vi "Bitte Warten.vi"() -> ()   [LabVIEW 2020, in "allgemeine Sub-VIs.lvlib"]
uses:
  allgemeine Sub-VIs.lvlib
  Visualisierungs Elemente/Button.ctl
  Aktionen Daten am cRIO speichern.ctl
  Sprachverwaltung/FGV Aktion Tabelle zerlegen.ctl
  SysLog/SysLog Interface.ctl
  SysLog/Aktionen FGV SysLog.ctl
  Sprachverwaltung/Sprachverwaltung.lvlib
  SysLog/SysLog.lvlib
panel:
  in  "Stopp":bool
  in  "gespeichert":bool
  out "String":string
  out "11":bool
  out "10":bool
  out "9":bool
  out "8":bool
  out "7":bool
  out "6":bool
  out "5":bool
  out "4":bool
  out "3":bool
  out "2":bool
  out "1":bool
  in  "Abbrechen":T1
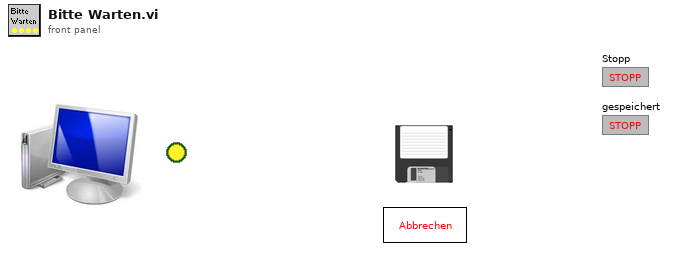
[diagram p1: front panel]
types:
  T1 = typedef "Button.ctl" = bool
  T2 = typedef "allgemeine Sub-VIs.lvlib/Aktionen Daten am cRIO speichern.ctl" = enum16{"lesen", "speichern setzen", "speichern reset", "gespeichert"}
  T3 = typedef "Sprachverwaltung.lvlib/FGV Aktion Tabelle zerlegen.ctl" = enum16{"laden", "vereinzeln", "speichern"}
  T4 = typedef "SysLog.lvlib/SysLog Interface.ctl" = cluster{"FehlermeldungsCode":i32, "ErfolgsmeldungsCode":i32, "ParameterListenString":string, "Anzeige":bool, "SysLogIcon":enum16{"OK", "Warnung", "Fehler"}, "intern":bool}
  T5 = typedef "SysLog.lvlib/Aktionen FGV SysLog.ctl" = enum16{"initialisieren", "lesen", "schreiben", "history button ref", "Syslog_Anforderung"}
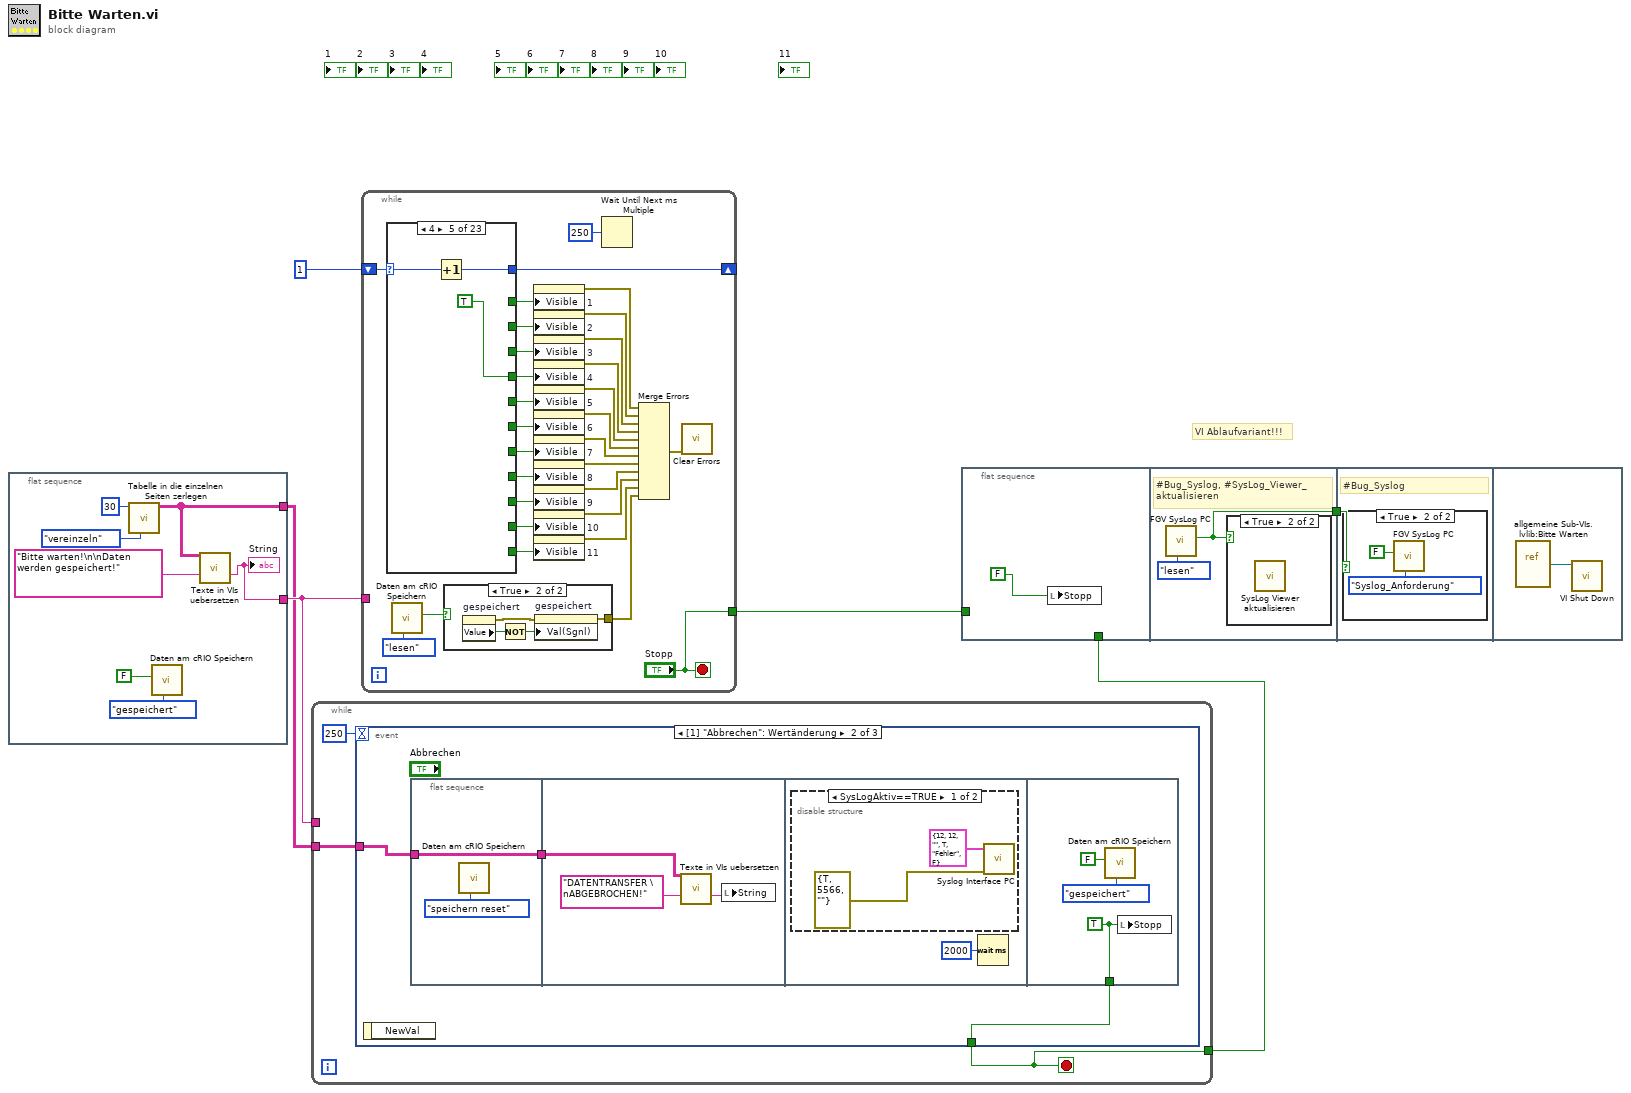
[diagram p0: block diagram]
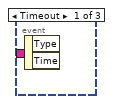
[diagram p4: hidden frame]
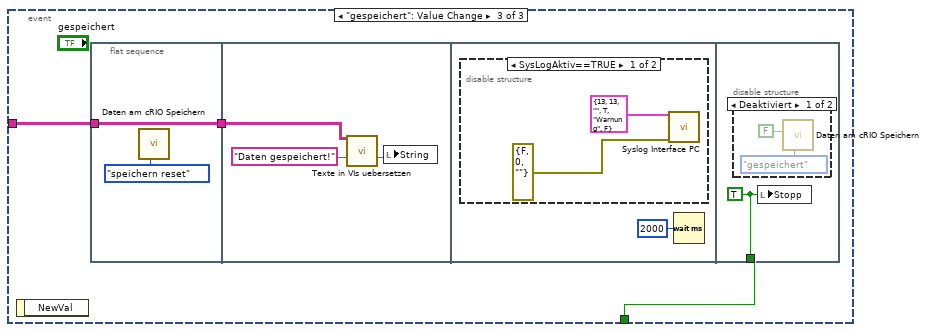
[diagram p6: hidden frame]
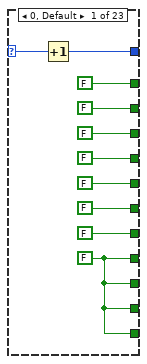
[diagram p10: hidden frame]
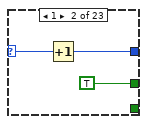
[diagram p11: hidden frame]
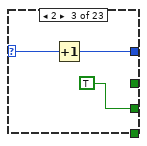
[diagram p12: hidden frame]
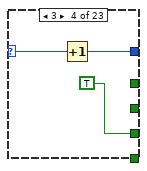
[diagram p13: hidden frame]
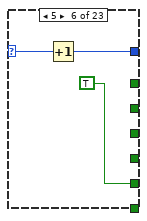
[diagram p14: hidden frame]
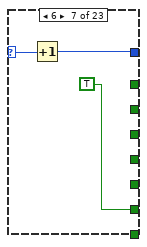
[diagram p15: hidden frame]
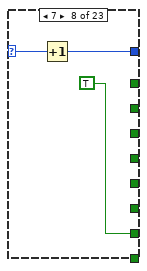
[diagram p16: hidden frame]
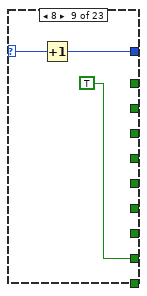
[diagram p17: hidden frame]
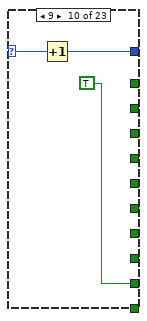
[diagram p18: hidden frame]
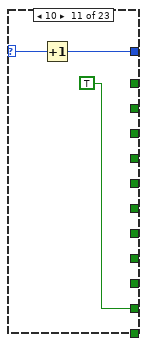
[diagram p19: hidden frame]
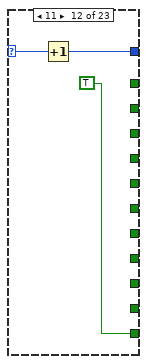
[diagram p20: hidden frame]
diagram:
  # "VI Ablaufvariant!!!"
  n1 = flat-sequence {
    tunnel: [w12] -> w5
    tunnel: [w10] -> w2
    frame #0 {
      n2 = call "Tabelle in die einzelnen Seiten zerlegen.vi"("Aktion"=FGV_Aktion_Tabelle_zerlegen."vereinzeln", "Index (Seite)"=30) -> ("Sprachliste"=w10:string[][])  [unwired: 7 in, 2 out]
      n3 = call "Daten am cRIO Speichern.vi"("Aktionen"=Aktionen_Daten_am_cRIO_speichern."gespeichert", "gespeichert"=FALSE) -> ()  [unwired: 8 in, 2 out]
      n4 = call "Texte in VIs uebersetzen.vi"("Sprachliste"=w10, "String zum Übersetzen"="Bitte warten!\n\nDaten werden gespeichert!" ("String")) -> ("String zum Übersetzen"=w12:string)  [unwired: 9 in, 4 out]
      "String" <- w12
    }
  }
  n5 = while {
    tunnel: w5 -> [_]
    tunnel: [w15] -> w3
    tunnel: w2 -> [w14]
    stop <- w15 stop-if-true
    n6 = event shown="[1] \"Abbrechen\": Wertänderung" {
      selector: _ -> [_ _ _]
      dyn-events: _ -> [_ _ _]
      timeout: 250 -> [_ _ _]
      tunnel: [_ w19 w33] -> w15
      tunnel: w14 -> [_ w17 w31]
      event Timeout {
        n7 = event-data() -> ()  [unwired: 1 in, 2 out]
      }
      event Value Change {
        n8 = event-data() -> ()  [unwired: 1 in, 1 out]
        n9 = flat-sequence {
          tunnel: w17 -> [w20]
          tunnel: [w20] -> w18
          tunnel: w18 -> [w22]
          tunnel: [w30] -> w19
          frame #0 {
            n10 = call "Daten am cRIO Speichern.vi"("Aktionen"=Aktionen_Daten_am_cRIO_speichern."speichern reset") -> ()  [unwired: 9 in, 2 out]
          }
          frame #1 {
            n11 = call "Texte in VIs uebersetzen.vi"("Sprachliste"=w22, "String zum Übersetzen"="DATENTRANSFER \nABGEBROCHEN!" ("String")) -> ("String zum Übersetzen"=w23:string)  [unwired: 9 in, 4 out]
            n12 = local write "String"(w23) -> ()
          }
          frame #2 {
            n13 = disable-structure shown="SysLogAktiv==TRUE" {
              frame condition #0 (active) {
                n14 = call "Syslog Interface PC.vi"("Fehler (in)"=errorcluster {"status"=TRUE, "code"=5566, "source"=""}, "Cluster (in)"=T4 {"FehlermeldungsCode"=12, "ErfolgsmeldungsCode"=12, "ParameterListenString"="", "Anzeige"=TRUE, "SysLogIcon"=enum."Fehler", "intern"=FALSE}) -> ()  [unwired: 9 in, 1 out]
              }
              frame condition #1 {
              }
            }
            n15 = Wait (ms)(milliseconds to wait=u32 2000 ("Zu wartende ms")) -> ()  [unwired: 1 out]
          }
          frame #3 {
            w30 = TRUE ("Stopp")
            n16 = call "Daten am cRIO Speichern.vi"("Aktionen"=Aktionen_Daten_am_cRIO_speichern."gespeichert", "gespeichert"=FALSE) -> ()  [unwired: 8 in, 2 out]
            n17 = local write "Stopp"(w30) -> ()
          }
        }
      }
      event "gespeichert": Value Change {
        n18 = event-data() -> ()  [unwired: 1 in, 1 out]
        n19 = flat-sequence {
          tunnel: [w34] -> w32
          tunnel: w31 -> [w34]
          tunnel: w32 -> [w36]
          tunnel: [w42] -> w33
          frame #0 {
            n20 = call "Daten am cRIO Speichern.vi"("Aktionen"=Aktionen_Daten_am_cRIO_speichern."speichern reset") -> ()  [unwired: 9 in, 2 out]
          }
          frame #1 {
            n21 = call "Texte in VIs uebersetzen.vi"("Sprachliste"=w36, "String zum Übersetzen"="Daten gespeichert!" ("String")) -> ("String zum Übersetzen"=w37:string)  [unwired: 9 in, 4 out]
            n22 = local write "String"(w37) -> ()
          }
          frame #2 {
            n23 = disable-structure shown="SysLogAktiv==TRUE" {
              frame condition #0 (active) {
                n24 = call "Syslog Interface PC.vi"("Fehler (in)"=errorcluster {"status"=FALSE, "code"=0, "source"=""}, "Cluster (in)"=T4 {"FehlermeldungsCode"=13, "ErfolgsmeldungsCode"=13, "ParameterListenString"="", "Anzeige"=TRUE, "SysLogIcon"=enum."Warnung", "intern"=FALSE}) -> ()  [unwired: 9 in, 1 out]
              }
              frame condition #1 {
              }
            }
            n25 = Wait (ms)(milliseconds to wait=u32 2000 ("Zu wartende ms")) -> ()  [unwired: 1 out]
          }
          frame #3 {
            w42 = TRUE ("Stopp")
            n26 = disable-structure shown="Deaktiviert" {
              frame Disabled {
                n27 = call "Daten am cRIO Speichern.vi"("Aktionen"=Aktionen_Daten_am_cRIO_speichern."gespeichert", "gespeichert"=FALSE) -> ()  [unwired: 8 in, 2 out]
              }
              frame Enabled {
              }
            }
            n28 = local write "Stopp"(w42) -> ()
          }
        }
      }
    }
  }
  n29 = while {
    shift-right: [w71] -> _
    shift-left: u8 1 -> [w72]
    tunnel: w5 -> [_]
    tunnel: ["Stopp"] -> w4
    stop <- "Stopp" stop-if-true
    n30 = case shown="4" w72 {
      selector: w72 -> [w88 w91 w93 w96 w99 w102 w105 w108 w111 w115 w118 w120 w124 w127 w130 w133 w136 w139 w142 w145 w147 w150 _]
      tunnel: [w87 w90 w92 w95 w98 w101 w104 w107 w110 w114 w117 w119 w123 w126 w129 w132 w135 w138 w141 w144 w146 w149 u8 1] -> w71
      tunnel: [FALSE TRUE _ _ _ _ _ _ _ _ _ _ TRUE _ _ _ _ _ _ _ _ _ _] -> w70
      tunnel: [w79 _ _ _ _ _ _ _ TRUE _ _ _ _ _ _ _ _ _ _ TRUE _ _ _] -> w69
      tunnel: [FALSE _ _ _ _ _ _ TRUE _ _ _ _ _ _ _ _ _ _ TRUE _ _ _ _] -> w68
      tunnel: [FALSE _ _ _ _ _ TRUE _ _ _ _ _ _ _ _ _ _ TRUE _ _ _ _ _] -> w67
      tunnel: [FALSE _ _ _ _ TRUE _ _ _ _ _ _ _ _ _ _ TRUE _ _ _ _ _ _] -> w66
      tunnel: [FALSE _ _ _ TRUE _ _ _ _ _ _ _ _ _ _ TRUE _ _ _ _ _ _ _] -> w65
      tunnel: [FALSE _ _ TRUE _ _ _ _ _ _ _ _ _ _ TRUE _ _ _ _ _ _ _ _] -> w64
      tunnel: [FALSE _ TRUE _ _ _ _ _ _ _ _ _ _ TRUE _ _ _ _ _ _ _ _ _] -> w63
      tunnel: [w79 _ _ _ _ _ _ _ _ _ _ TRUE _ _ _ _ _ _ _ _ _ _ TRUE] -> w62
      tunnel: [w79 _ _ _ _ _ _ _ _ _ TRUE _ _ _ _ _ _ _ _ _ _ TRUE _] -> w61
      tunnel: [w79 _ _ _ _ _ _ _ _ TRUE _ _ _ _ _ _ _ _ _ _ TRUE _ _] -> w60
      frame 0, Default {
        w79 = FALSE
        n31 = Increment(x=w88) -> (x+1=w87:u8)
      }
      frame 1 {
        n32 = Increment(x=w91) -> (x+1=w90:u8)
      }
      frame 2 {
        n33 = Increment(x=w93) -> (x+1=w92:u8)
      }
      frame 3 {
        n34 = Increment(x=w96) -> (x+1=w95:u8)
      }
      frame 4 {
        n35 = Increment(x=w99) -> (x+1=w98:u8)
      }
      frame 5 {
        n36 = Increment(x=w102) -> (x+1=w101:u8)
      }
      frame 6 {
        n37 = Increment(x=w105) -> (x+1=w104:u8)
      }
      frame 7 {
        n38 = Increment(x=w108) -> (x+1=w107:u8)
      }
      frame 8 {
        n39 = Increment(x=w111) -> (x+1=w110:u8)
      }
      frame 9 {
        n40 = Increment(x=w115) -> (x+1=w114:u8)
      }
      frame 10 {
        n41 = Increment(x=w118) -> (x+1=w117:u8)
      }
      frame 11 {
        n42 = Increment(x=w120) -> (x+1=w119:u8)
      }
      frame 12 {
        n43 = Increment(x=w124) -> (x+1=w123:u8)
      }
      frame 13 {
        n44 = Increment(x=w127) -> (x+1=w126:u8)
      }
      frame 14 {
        n45 = Increment(x=w130) -> (x+1=w129:u8)
      }
      frame 15 {
        n46 = Increment(x=w133) -> (x+1=w132:u8)
      }
      frame 16 {
        n47 = Increment(x=w136) -> (x+1=w135:u8)
      }
      frame 17 {
        n48 = Increment(x=w139) -> (x+1=w138:u8)
      }
      frame 18 {
        n49 = Increment(x=w142) -> (x+1=w141:u8)
      }
      frame 19 {
        n50 = Increment(x=w145) -> (x+1=w144:u8)
      }
      frame 20 {
        n51 = Increment(x=w147) -> (x+1=w146:u8)
      }
      frame 21 {
        n52 = Increment(x=w150) -> (x+1=w149:u8)
      }
      frame 22 {
      }
    }
    n53 = call "Daten am cRIO Speichern.vi"("Aktionen"=Aktionen_Daten_am_cRIO_speichern."lesen") -> ("gespeichert"=w59:bool)  [unwired: 9 in, 1 out]
    n54 = case shown="True" w59 {
      tunnel: [_ w75] -> w46
      frame False {
      }
      frame True {
        n55 = property on="gespeichert" class="Bool. (strikt)"() -> (error out=w76:errorcluster, "Value"=w77:bool)  [unwired: 2 in, 1 out]
        n56 = Not(x=w77) -> (.not. x?=w78:bool)
        n57 = property on="gespeichert" class="Bool. (strikt)"(error in=w76, "Val(Sgnl)"=w78) -> (error out=w75:errorcluster)  [unwired: 1 in, 1 out]
      }
    }
    n58 = property on="1" class="Bool. (strikt)"("Visible"=w70) -> (error out=w57:errorcluster)  [unwired: 2 in, 1 out]
    n59 = property on="2" class="Bool. (strikt)"("Visible"=w63) -> (error out=w56:errorcluster)  [unwired: 2 in, 1 out]
    n60 = property on="3" class="Bool. (strikt)"("Visible"=w64) -> (error out=w55:errorcluster)  [unwired: 2 in, 1 out]
    n61 = property on="4" class="Bool. (strikt)"("Visible"=w65) -> (error out=w54:errorcluster)  [unwired: 2 in, 1 out]
    n62 = property on="5" class="Bool. (strikt)"("Visible"=w66) -> (error out=w53:errorcluster)  [unwired: 2 in, 1 out]
    n63 = property on="6" class="Bool. (strikt)"("Visible"=w67) -> (error out=w52:errorcluster)  [unwired: 2 in, 1 out]
    n64 = property on="7" class="Bool. (strikt)"("Visible"=w68) -> (error out=w51:errorcluster)  [unwired: 2 in, 1 out]
    n65 = property on="8" class="Bool. (strikt)"("Visible"=w69) -> (error out=w50:errorcluster)  [unwired: 2 in, 1 out]
    n66 = property on="9" class="Bool. (strikt)"("Visible"=w60) -> (error out=w49:errorcluster)  [unwired: 2 in, 1 out]
    n67 = property on="10" class="Bool. (strikt)"("Visible"=w61) -> (error out=w48:errorcluster)  [unwired: 2 in, 1 out]
    n68 = property on="11" class="Bool. (strikt)"("Visible"=w62) -> (error out=w47:errorcluster)  [unwired: 2 in, 1 out]
    n69 = Wait Until Next ms Multiple(millisecond multiple=u32 250 ("Vielfache von ms")) -> ()  [unwired: 1 out]
    n70 = Merge Errors(w57, w56, w55, w54, w53, w52, w51, w50, w49, w48, w47, w46) -> (w45:errorcluster)
    n71 = call <vilib>:"Clear Errors.vi"("error in (no error)"=w45) -> ()  [unwired: 5 in, 2 out]
  }
  n72 = flat-sequence {
    tunnel: w4 -> [_]
    tunnel: w3 -> [_]
    tunnel: [w155] -> w1
    tunnel: w1 -> [w157]
    frame #0 {
      n73 = local write "Stopp"(FALSE ("gespeichert")) -> ()
    }
    frame #1 {
      # "#Bug_Syslog, #SysLog_Viewer_aktualisieren"
      n74 = call "FGV SysLog PC.vi"("Aktion"=Aktionen_FGV_SysLog."lesen") -> ("Syslog Anforderung"=w155:bool)  [unwired: 6 in, 4 out]
      n75 = case shown="True" w155 {
        frame False {
        }
        frame True {
          n76 = call "SysLog Viewer aktualisieren.vi"() -> ()  [unwired: 12 in]
        }
      }
    }
    frame #2 {
      # "#Bug_Syslog"
      n77 = case shown="True" w157 {
        frame False {
        }
        frame True {
          n78 = call "FGV SysLog PC.vi"("Aktion"=Aktionen_FGV_SysLog."Syslog_Anforderung", "Syslog Anforderung"=T1 FALSE ("SysLogHistory")) -> ()  [unwired: 5 in, 5 out]
        }
      }
    }
    frame #3 {
      n79 = vi-ref "allgemeine Sub-VIs.lvlib:Bitte Warten.vi"() -> (w160:refnum<vi>)
      n80 = call "VI Shut Down.vi"("VI Referenz"=w160) -> ()  [unwired: 11 in]
    }
  }
